vi "global_vars.vi"() -> ()   [LabVIEW 2011]
uses:
  <vilib>/userdefined/High Color/IMAQdx.ctl
panel:
  in  "dbl_shutter_value":dbl=0.036604516208171844 min=0.001 max=1.0
  in  "df_intial phase shift":dbl
  in  "df_#fringes":dbl=4.0 caption="#fringes"
  out "ul_ar_pxar_capt_images":u8[][][](array[numeric])
  out "ul_ar_pxar_orig_patterns":u8[][][](array[numeric])
  in  "ID_camera_in_Use":T1="HP Webcam"
  out "Image_Type":T2 items=["Grayscale (U8)", "Grayscale (I16)", "Grayscale (SGL)", "Complex (CSG)", "RGB (U32)", "HSL (U32)", "RGB (U64)", "Grayscale (U16)"]
  in  "UL_#Phase Shifts":i32=4
  in  "I32_clu_window_size":cluster{"x Width(Px)":i32, "y height(Px)":i32}={"x Width(Px)"=500, "y height(Px)"=500}
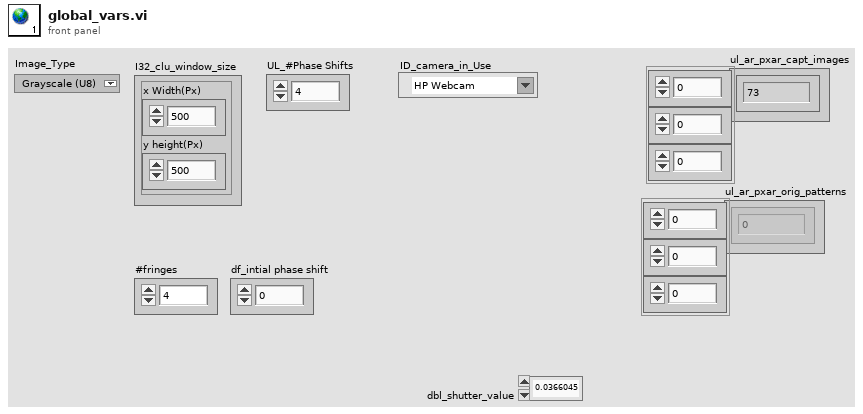
[diagram p1: front panel]
types:
  T1 = typedef "IMAQdx.ctl" = refnum<k21>
  T2 = typedef "Image Type" = u32
diagram:
